vi "Simulator PWM Config Test.vi"(4 "error in (no error)":errorcluster, 6 "Configuration":T1={"BusType"=enum."GPIB", "GPIB Bus"=0, "GPIB Address"=22, "IP"=0, "COM"=1, "Baud Rate"=enum."9600"}, 7 "Str Refnum":refnum<vi>) -> (0 "error out":errorcluster)   [LabVIEW 2011]
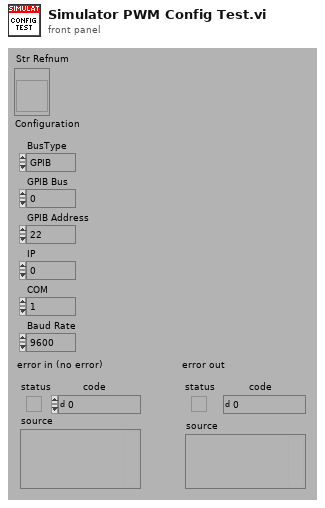
[diagram p1: front panel]
types:
  T1 = cluster{"BusType":enum32{"GPIB", "LAN/IP", "Serial"}, "GPIB Bus":i32, "GPIB Address":i32, "IP":u32, "COM":i32, "Baud Rate":enum16{"300", "600", "1200", "2400", "4800", "9600"}}
  T2 = enum16{"300", "600", "1200", "2400", "4800", "9600"}
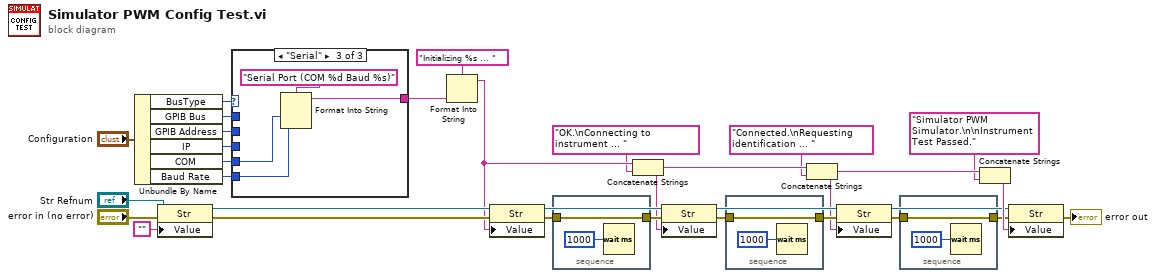
[diagram p0: block diagram]
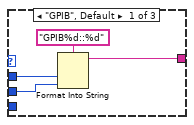
[diagram p2: hidden frame]
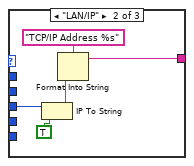
[diagram p3: hidden frame]
diagram:
  n1 = Unbundle By Name("Configuration") -> ("BusType"=w25:enum32{"GPIB", "LAN/IP", "Serial"}, "GPIB Bus"=w24:i32, "GPIB Address"=w23:i32, "IP"=w22:u32, "COM"=w21:i32, "Baud Rate"=w1:T2)
  n2 = property class="Str"(reference="Str Refnum", error in="error in (no error)", "Value"="") -> (reference out=w18:refnum<vi>, error out=w28:errorcluster)
  n3 = case shown="\"Serial\"" w25 {
    tunnel: w24 -> [w34 _ _]
    tunnel: w23 -> [w33 _ _]
    tunnel: w22 -> [_ w39 _]
    tunnel: w21 -> [_ _ w43]
    tunnel: [w32 w36 w42] -> w20
    tunnel: w1 -> [_ _ w41]
    frame "GPIB", Default {
      n4 = Format Into String(format string="GPIB%d::%d", w34, w33) -> (resulting string=w32:string)  [unwired: 2 in, 1 out]
    }
    frame "LAN/IP" {
      n5 = IP To String(1:TRUE, 2:w39) -> (0:w38:string)
      n6 = Format Into String(format string="TCP/IP Address %s", w38) -> (resulting string=w36:string)  [unwired: 2 in, 1 out]
    }
    frame "Serial" {
      n7 = Format Into String(format string="Serial Port (COM %d Baud %s)", w43, w41) -> (resulting string=w42:string)  [unwired: 2 in, 1 out]
    }
  }
  n8 = Format Into String(format string="Initializing %s ... ", w20) -> (resulting string=w11:string)  [unwired: 2 in, 1 out]
  n9 = property class="Str"(reference=w18, error in=w28, "Value"=w11) -> (reference out=w16:refnum<vi>, error out=w19:errorcluster)
  n10 = stacked-sequence {
    tunnel: w19 -> [w45]
    tunnel: [w45] -> w17
    frame #0 {
      n11 = Wait (ms)(milliseconds to wait=u32 1000) -> ()  [unwired: 1 out]
    }
  }
  n12 = Concatenate Strings(w11, "OK.\nConnecting to instrument ... ") -> (w9:string)
  n13 = property class="Str"(reference=w16, error in=w17, "Value"=w9) -> (reference out=w13:refnum<vi>, error out=w15:errorcluster)
  n14 = stacked-sequence {
    tunnel: w15 -> [w47]
    tunnel: [w47] -> w14
    frame #0 {
      n15 = Wait (ms)(milliseconds to wait=u32 1000) -> ()  [unwired: 1 out]
    }
  }
  n16 = Concatenate Strings(w9, "Connected.\nRequesting identification ... ") -> (w5:string)
  n17 = property class="Str"(reference=w13, error in=w14, "Value"=w5) -> (reference out=w2:refnum<vi>, error out=w12:errorcluster)
  n18 = stacked-sequence {
    tunnel: w12 -> [w49]
    tunnel: [w49] -> w6
    frame #0 {
      n19 = Wait (ms)(milliseconds to wait=u32 1000) -> ()  [unwired: 1 out]
    }
  }
  n20 = Concatenate Strings(w5, "Simulator PWM Simulator.\n\nInstrument Test Passed.") -> (w7:string)
  n21 = property class="Str"(reference=w2, error in=w6, "Value"=w7) -> (error out=→"error out":errorcluster)  [unwired: 1 out]
